vi "Sort Coincs by top or bottom.vi"(3 "Coincs":T1[](array[typedef])) -> (0 "Bottom Coincs":T1[](array[typedef]), 1 "Top Coincs":T1[](array[typedef]))   [LabVIEW 2016]
uses:
  Typedefs/Coincidence.ctl
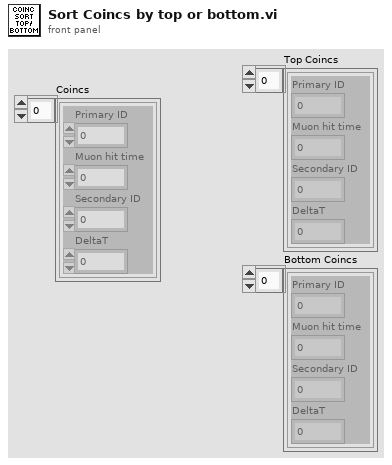
[diagram p1: front panel]
types:
  T1 = typedef "Coincidence.ctl" = cluster{"Primary ID":i8, "Muon hit time":u64, "Secondary ID":i8, "DeltaT":i32}
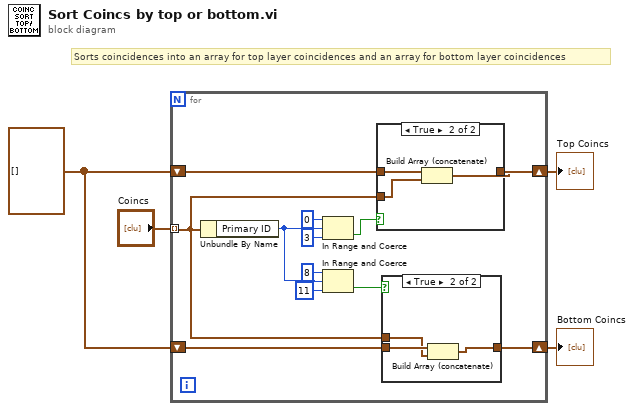
[diagram p0: block diagram]
diagram:
  w3 = T1[] []
  # "Sorts coincidences into an array for top layer coincidences and an array for bottom layer coincidences"
  n1 = for {
    tunnel: "Coincs" -> [w6] mode=indexing
    shift-right: [w9] -> w2
    shift-left: w3 -> [w8]
    shift-right: [w5] -> w1
    shift-left: w3 -> [w7]
    n2 = Unbundle By Name(w6) -> ("Primary ID"=w11:i8)
    n3 = In Range and Coerce(upper limit=i8 0, x=w11, lower limit=i8 3) -> (In Range?=w14:bool)  [unwired: 1 out]
    n4 = In Range and Coerce(upper limit=i8 8, x=w11, lower limit=i8 11) -> (In Range?=w10:bool)  [unwired: 1 out]
    n5 = case shown="True" w14 {
      tunnel: w6 -> [_ w24]
      tunnel: [w21 w23] -> w9
      tunnel: w8 -> [w21 w22]
      frame False {
      }
      frame True {
        n6 = Build Array (concatenate)(w22, w24) -> (w23:T1[])
      }
    }
    n7 = case shown="True" w10 {
      tunnel: w7 -> [w17 w20]
      tunnel: w6 -> [_ w19]
      tunnel: [w17 w18] -> w5
      frame False {
      }
      frame True {
        n8 = Build Array (concatenate)(w20, w19) -> (w18:T1[])
      }
    }
  }
  "Top Coincs" <- w2
  "Bottom Coincs" <- w1
